vi "例4-24.vi"() -> ()   [LabVIEW 2019]
uses:
  <vilib>/Analysis/NI_AALBase.lvlib
panel:
  out "记录时间":string
  out "记录波形":dbl[](graph)
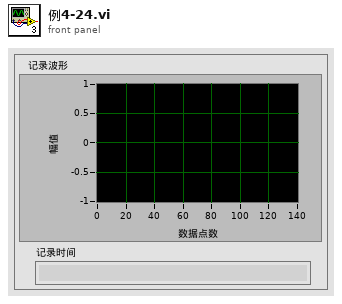
[diagram p1: front panel]
types:
  T1 = enum16{"open", "replace", "create", "open or create", "replace or create", "replace or create with confirmation"}
  T2 = cluster{"date/time string":string, "sine wave":dbl[]}
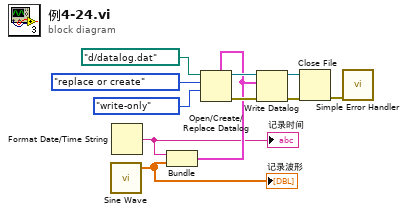
[diagram p0: block diagram]
diagram:
  n1 = call <vilib>:"Sine Wave.vi"() -> ("sine wave"=w1:dbl[])  [unwired: 5 in, 2 out]
  "记录波形" <- w1
  n2 = Format Date/Time String() -> (date/time string=w2:string)  [unwired: 3 in]
  "记录时间" <- w2
  n3 = Bundle("date/time string"=w2, "sine wave"=w1) -> (w5:T2)  [unwired: 1 in]
  n4 = Open/Create/Replace Datalog(5:w5, 9:enum16{"read/write", "read-only", "write-only"}."write-only" ("权限(0:read/write)"), 10:T1."replace or create" ("操作(0:open)"), 11:path "d:/datalog.dat" ("数据记录路径（使用对话框）")) -> (0:w6:errorcluster, 3:w7:refnum<k1>)  [unwired: 2 in, 1 out]
  n5 = Write Datalog(4:w6, 6:w5, 7:w7) -> (0:w3:errorcluster, 3:w4:refnum<k1>)
  n6 = Close File(refnum=w4, error in=w3) -> (error out=w11:errorcluster)  [unwired: 1 out]
  n7 = call <vilib>:"Simple Error Handler.vi"("error in (no error)"=w11) -> ()  [unwired: 4 in, 5 out]
